vi "Digital_Bridge_3_kart.vi"() -> ()   [LabVIEW 2014]
uses:
  <vilib>/Utility/error.llb/DialogType.ctl
  <vilib>/DAQmx/write.llb/DAQmx Write (Analog 1D Wfm NChan NSamp).vi
  DB_Global_4_kart-Test.vi
  <vilib>/DAQmx/create/channels.llb/DAQmx Create Channel (AO-Voltage-Basic).vi
  <vilib>/DAQmx/configure/timing.llb/DAQmx Timing (Sample Clock).vi
  <vilib>/DAQmx/create/channels.llb/DAQmx Create Channel (AI-Voltage-Basic).vi
  <vilib>/DAQmx/configure/trigger.llb/DAQmx Start Trigger (Digital Edge).vi
  <vilib>/DAQmx/miscellaneous.llb/DAQmx Fill In Error Info.vi
  Sub_VI/show_sensitivity.vi
  First_input_values.vi
  <resource>/objmgr/daqmx.rc
  <vilib>/measure/NI_MABase.lvlib
panel:
  out "input values 2":dbl[](array[numeric])
  out "Y Range KV":dbl
  out "Y Range W":dbl
  out "Y Range 1R":dbl
  out "Y Range 10R":dbl
  out "Y Range AD":dbl
  out "Y 2.input KV":dbl
  out "Y 2.input W":dbl
  out "Y 2.input 1R":dbl
  out "Y 2.input 10R":dbl
  out "Y 2.input AD":dbl
  out "Y 1.input KV":dbl
  out "Y 1.input W":dbl
  out "Y 1.input 1R":dbl
  out "Y 1.input 10R":dbl
  out "Y 1.input AD":dbl
  out "X Range KV":dbl
  out "X Range W":dbl
  out "X Range 1R":dbl
  out "X Range 10R":dbl
  out "X Range AD":dbl
  out "X 2.input KV":dbl
  out "X 2.input W":dbl
  out "X 2.input 1R":dbl
  out "X 2.input 10R":dbl
  out "X 2.input AD":dbl
  out "X 1.input KV":dbl
  out "X 1.input W":dbl
  out "X 1.input 1R":dbl
  out "X 1.input 10R":dbl
  out "X 1.input AD":dbl
  in  "Open all":bool
  in  "Kelvin":bool
  in  "Wagner":bool
  in  "1R":bool
  in  "10R":bool
  in  "AD":bool
  out "count meas":u16
  out "cycle 10r 1r":bool[](array[boolean])
  out "dummy fix default":bool
  out "1 or 10":i32
  in  "read x1 y1":bool
  in  "read x2 y2":bool
  in  "result phase":bool
  in  "read x1 y1 2":bool
  in  "read x2 y2 2":bool
  in  "result phase 2":bool
  in  "read x1 y1 3":bool
  in  "read x2 y2 3":bool
  in  "result phase 3":bool
  in  "read x1 y1 5":bool
  in  "read x2 y2 5":bool
  in  "result phase 5":bool
  in  "result phase 4":bool
  in  "Output Y2":dbl
  in  "Output X2":dbl
  in  "Output Y1":dbl
  in  "Output X1":dbl
  in  "read x2 y2 4":bool
  in  "read x1 y1 4":bool
  in  "Contiune AD":bool
  in  "Contiune Kelvin":bool
  in  "Contiune Wagner":bool
  in  "Contiune 1R":bool
  in  "Contiune 10R":bool
  out "error 2":bool
  out "Outpu Denge Kosulu y1_y2":dbl[][](array[numeric])
  out "Output Denge Kosulu x1_x2":dbl[][](array[numeric])
  out "Output Denge Kosulu x2_y2":dbl[][](array[numeric])
  in  "fix default":bool
  in  "Cluster 2":T1
  in  "Cluster":T2
  out "input values":dbl[](array[numeric])
  out "stop listbox":bool
  out "F Values Array":dbl[][](array[numeric])
  out "extra default values":dbl[][](array[numeric])
  out "control hz array":dbl[][](array[numeric])
  out "Frekanslar":dbl[](array[numeric])
  out "Denge Kosulu y1_y2":dbl[][](array[numeric])
  out "Denge Kosulu x1_x2":dbl[][](array[numeric])
  out "Denge Kosulu x2_y2":dbl[][](array[numeric])
  out "Other Boolean Array":bool[](array[boolean])
  out "Other Array":dbl[](array[numeric])
  out "Kelvin F/P Array":dbl[][](array[numeric])
  out "Wagner F/P Array":dbl[][](array[numeric])
  out "1R F/P Array":dbl[][](array[numeric])
  out "10R F/P Array":dbl[][](array[numeric])
  out "AD F/P Array":dbl[][](array[numeric])
  in  "default input":bool
  out "pass hz":bool
  in  "continue":bool
  out "default values":T3(array[cluster]) {"Kelvin Yk-1" format="%.4p"; "Wagner Yk-1" format="%.4p"; "1R Yk-1" format="%.4p"; "10R Yk-1" format="%.4p"; "Ana Denge Yk-1" format="%.4p"; "Kelvin Yk" format="%.4p"; "Wagner Yk" format="%.4p"; "1R Yk" format="%.4p"; "10R Yk" format="%.4p"; "Ana Denge Yk" format="%.4p"; "Kelvin Xk-1" format="%.4p"; "Wagner Xk-1" format="%.4p"; "1R Xk-1" format="%.4p"; "10R Xk-1" format="%.4p"; "Ana Denge Xk-1" format="%.4p"; "Kelvin Xk" format="%.4p"; "Wagner Xk" format="%.4p"; "1R Xk" format="%.4p"; "10R Xk" format="%.4p"; "Ana Denge Xk" format="%.4p"}
  out "frekans index":dbl
  in  "Direnc 1 [ohm]":dbl=10000.0
  in  "Direnc 2 [ohm]":dbl=1000.0
  in  "error":bool
  out "iterasyon AD":dbl=1.0
  out "first process":bool
  out "reset values":bool
  out "finish":bool
  out "end time":string
  out "start time":string
  out "Iterasyon Successful":dbl
  in  "RESET SENS Y":bool
  in  "RESET SENS X":bool
  in  "RESET SENS Y 5":bool
  in  "RESET SENS X 5":bool
  in  "RESET SENS Y 3":bool
  in  "RESET SENS X 3":bool
  in  "RESET SENS Y 2":bool
  in  "RESET SENS X 2":bool
  in  "RESET SENS Y 4":bool
  in  "RESET SENS X 4":bool
  in  "Activate":bool
  in  "Denge Kolu":u16(ring) items=["Default", "Ana Denge", "Wagner", "10R", "1R"]
  in  "Yedek Kart offset":dbl caption="Offset"
  in  "SWITCH":bool
  in  "Mux2":u16(ring) items=["Wagner", "Ground"]
  in  "Mux1":u16(ring) items=["Open All", "Ana Denge", "10R", "1R"]
  in  "Stop":bool
  in  "GPIB In":refnum<visa-resource-name>="GPIB0::8::INSTR"
  in  "Reference Phase (0.000 degrees)":string
  in  "REFERANS FAZ":bool
  in  "Input Source (0: A)":u16(ring) items=["A", "A-B"]
  in  "INPUT SOURCE":bool
  in  "Sensitivity":u16(ring)=13 items=["2 nV", "5 nV", "10 nV", "20 nV", "50 nV", "100 nV", "200 nV", "500 nV", "1 uV", "2 uV", "5 uV", "10 uV", "20 uV", "50 uV", "100 uV", "200 uV", "500 uV", "1mV", "2 mV", "5 mV", "10 mV", "20 mV", "50 mV", "100 mV", "200 mV", "500 mV", "1 V"]
  in  "SENSITIVITY":bool
  in  "Tab Control":T4(tab)=enum."Wagner"
  in  "Manuel Input":bool
  in  "delay s":u32=2 min=1 max=100
  in  "delay f":u32=2 min=1 max=100
  in  "set":u16=1 min=1 max=100
  in  "BASLAT":bool
  in  "Denge Seçimi":u8=4 min=1 max=5
  in  "Manuel/Otomatik":enum16{"Manuel", "Otomatik"}(ring)=enum."Otomatik"
  out "Hatalar":string[](array[string])
  in  "olcum":u16=1 min=1 max=100
  in  "Frekans Listbox":i32[](listbox)=[12]
  in  "Default Values Listbox":i32[](listbox)=[4]
  in  "Direnc 1 - Direnc 2":u32(ring)=2 items=["1M(Ohm) / 100K(Ohm)", "100K(Ohm) / 10K(Ohm)", "10K(Ohm) / 1K(Ohm)", "1K(Ohm) / 100(Ohm)", "100(Ohm) / 10(Ohm)", "10(Ohm) / 1(Ohm)", "1M(Ohm) / 1M(Ohm)", "100K(Ohm) / 100K(Ohm)", "10K(Ohm) / 10K(Ohm)", "1K(Ohm) / 1K(Ohm)", "100(Ohm) / 100(Ohm)", "10(Ohm) / 10(Ohm)", "1(Ohm) / 1(Ohm)", "1000nF / 100nF (CP)", "100nF / 10nF (CP)", "10nF / 1nF (CP)", "1nF / 100pF (CP)", "100pF / 10pF (CP)", "10pF / 1pF (CP)", "1000nF / 1000nF (CP)", "100nF / 100nF (CP)", "10nF / 10nF (CP)", "1nF / 1nF (CP)", "100pF / 100pF (CP)", "10pF / 10pF (CP)", "1pF / 1pF (CP)"]
  in  "Multicolumn Listbox":i32(listbox)
  in  "Cp - 10R":u16(ring) items=["1nF", "10nF", "100nF", "1uF", "10uF"]
  in  "Cp - 1R":u16(ring) items=["1nF", "10nF", "100nF", "1uF", "10uF"]
  in  "value 10R":u16
  in  "value 1R":u16
  in  "Sheet name":string="10k1k"
  in  "Manuel Setup":bool
  in  "interrupt":bool=TRUE
  in  "START X":bool
  in  "START Y":bool
  out "AD X(k-1)":dbl=0.01
  out "AD Xk":dbl
  out "AD Yk":dbl
  out "AD Y(k-1)":dbl=0.01
  in  "AD X_1":dbl=3e-06
  in  "AD X_2":dbl=4e-07
  in  "AD Y_1":dbl=3e-06
  in  "AD Y_2":dbl=4e-07
  out "İterasyon X":dbl
  out "İterasyon Y":dbl
  in  "X":bool
  in  "X1":bool
  in  "RANGE KONTROL X":bool
  in  "IF ELSE X":bool
  in  "KONTROL Y":bool
  out "result output x [AD]":dbl
  out "output 2 x [ana denge]":dbl
  out "output 1 x [ana denge]":dbl
  out "input 1 x [ana denge]":dbl format="%.4p"
  out "input 2 x [ana denge]":dbl format="%.4p"
  in  "Y1":bool
  in  "Y":bool
  in  "IF ELSE Y":bool
  in  "RANGE KONTROL Y":bool
  in  "KONTROL X":bool
  out "result output y [AD]":dbl
  out "input 1 y [ana denge]":dbl format="%.4p"
  out "input 2 y [ana denge]":dbl format="%.4p"
  out "output 1 y [ana denge]":dbl
  out "output 2 y [ana denge]":dbl
  in  "PASS ANA D":bool
  out "Boolean":bool
  in  "Ana denge Switch":bool
  in  "Start AD Y":bool
  in  "Start AD X":bool
  in  "auto phase AD":bool
  in  "Reserve AD":u16(ring) items=["Max", "Manuel", "Min"]
  in  "Optimum Range 1":bool
  in  "START X 2":bool
  in  "START Y 2":bool
  out "İterasyon Y 2":dbl
  out "İterasyon X 2":dbl
  out "10R Y(k-1)":dbl=3.0
  out "10R Yk":dbl
  out "10R X(k-1)":dbl=3.0
  out "10R Xk":dbl
  in  "10R  Y_1":dbl=4e-05
  in  "10R X_1":dbl=4e-05
  in  "10R Y_2":dbl=2e-05
  in  "10R X_2":dbl=2e-05
  in  "X 2":bool
  in  "X1 2":bool
  in  "RANGE KONTROL X 2":bool
  in  "IF ELSE X 2":bool
  in  "KONTROL Y 2":bool
  out "result output x [10R]":dbl
  out "output 2 x [10R]":dbl
  out "output 1 x [10R]":dbl
  out "input 1 x [10R]":dbl format="%.4p"
  out "input 2 x [10R]":dbl format="%.4p"
  in  "Y 2":bool
  in  "Y1 2":bool
  in  "IF ELSE Y 2":bool
  in  "RANGE KONTROL Y 2":bool
  in  "KONTROL X 2":bool
  out "result output y [10R]":dbl
  out "input 1 y [10R]":dbl format="%.4p"
  out "input 2 y [10R]":dbl format="%.4p"
  out "output 1 y [10R]":dbl
  out "output 2 y [10R]":dbl
  in  "PASS 10R":bool
  in  "10R switch":bool
  in  "Start 10R Y":bool
  in  "Start 10R X":bool
  out "Boolean 2":bool
  in  "auto phase 10R":bool
  in  "Reserve 10R":u16(ring) items=["Max", "Manuel", "Min"]
  in  "Optimum Range 2":bool
  in  "START X 3":bool
  in  "START Y 3":bool
  out "İterasyon Y 3":dbl
  out "İterasyon X 3":dbl
  out "1R Y(k-1)":dbl=2.0
  out "1R Yk":dbl
  out "1R X(k-1)":dbl=2.0
  out "1R Xk":dbl
  in  "1R Y_1":dbl=4e-05
  in  "1R X_1":dbl=4e-05
  in  "1R Y_2":dbl=2e-05
  in  "1R X_2":dbl=2e-05
  in  "X 3":bool
  in  "X1 3":bool
  in  "RANGE KONTROL X 3":bool
  in  "IF ELSE X 3":bool
  in  "KONTROL Y 3":bool
  out "result output x [1R]":dbl
  out "output 2 x [1R]":dbl
  out "output 1 x [1R]":dbl
  out "input 1 x [1R]":dbl format="%.4p"
  out "input 2 x [1R]":dbl format="%.4p"
  in  "Y 3":bool
  in  "Y1 3":bool
  in  "IF ELSE Y 3":bool
  in  "RANGE KONTROL Y 3":bool
  in  "KONTROL X 3":bool
  out "result output y [1R]":dbl
  out "input 1 y [1R]":dbl format="%.4p"
  out "input 2 y [1R]":dbl format="%.4p"
  out "output 1 y [1R]":dbl
  out "output 2 y [1R]":dbl
  in  "PASS 1R":bool
  in  "1R switch":bool
  in  "Start 1R Y":bool
  in  "Start 1R X":bool
  out "Boolean 3":bool
  in  "auto phase 1R":bool
  in  "Reserve 1R":u16(ring) items=["Max", "Manuel", "Min"]
  in  "Optimum Range 3":bool
  in  "START X 4":bool
  in  "START Y 4":bool
  out "İterasyon Y 4":dbl
  out "İterasyon X 4":dbl
  out "Wagner Y(k-1)":dbl=0.1
  out "Wagner Yk":dbl
  out "Wagner  X(k-1)":dbl=0.1
  out "Wagner Xk":dbl
  in  "Wagner Y_1":dbl=5e-05
  in  "Wagner X_1":dbl=5e-05
  in  "Wagner Y_2":dbl=2e-05
  in  "Wagner X_2":dbl=2e-05
  out "result output x [Wagner]":dbl
  out "output 2 x [wagner]":dbl
  out "output 1 x [wagner]":dbl
  in  "X 4":bool
  in  "X1 4":bool
  out "input 1 x [wagner]":dbl format="%.4p"
  out "input 2 x [wagner]":dbl format="%.4p"
  in  "RANGE KONTROL X 4":bool
  in  "IF ELSE X 4":bool
  in  "KONTROL Y 4":bool
  in  "PASS WAGNER":bool
  out "result output y [Wagner]":dbl
  out "input 1 y [wagner]":dbl format="%.4p"
  out "input 2 y [wagner]":dbl format="%.4p"
  out "output 1 y [wagner]":dbl
  out "output 2 y [wagner]":dbl
  in  "IF ELSE Y 4":bool
  in  "RANGE KONTROL Y 4":bool
  in  "Y 4":bool
  in  "Y1 4":bool
  in  "KONTROL X 4":bool
  in  "wagner switch":bool
  in  "Start Wagner Y":bool
  in  "Start Wagner X":bool
  out "Boolean 4":bool
  in  "auto phase wagner":bool
  in  "Reserve Wagner":u16(ring) items=["Max", "Manuel", "Min"]
  in  "Optimum Range 4":bool
  in  "START X 5":bool
  in  "START Y 5":bool
  out "İterasyon Y 5":dbl
  out "İterasyon X 5":dbl
  out "Kelvin Y(k-1)":dbl=0.01
  out "Kelvin Yk":dbl
  out "Kelvin X(k-1)":dbl=0.01
  out "Kelvin Xk":dbl
  in  "Kelvin Y_1":dbl=3e-06
  in  "Kelvin X_1":dbl=3e-06
  in  "Kelvin Y_2":dbl=2e-07
  in  "Kelvin X_2":dbl=2e-07
  in  "X 5":bool
  in  "X1 5":bool
  in  "RANGE KONTROL X 5":bool
  in  "IF ELSE X 5":bool
  in  "KONTROL Y 5":bool
  out "result output x [Kelvin]":dbl
  out "output 2 x [kelvin]":dbl
  out "output 1 x [kelvin]":dbl
  out "input 1 x [kelvin]":dbl format="%.4p"
  out "input 2 x [kelvin]":dbl format="%.4p"
  in  "Y 5":bool
  in  "Y1 5":bool
  in  "IF ELSE Y 5":bool
  in  "RANGE KONTROL Y 5":bool
  in  "KONTROL X 5":bool
  out "result output y [Kelvin]":dbl
  out "input 1 y [kelvin]":dbl format="%.4p"
  out "input 2 y [kelvin]":dbl format="%.4p"
  out "output 1 y [kelvin]":dbl
  out "output 2 y [kelvin]":dbl
  in  "PASS KELVIN":bool
  in  "kelvin switch":bool
  in  "Start Kelvin Y":bool
  in  "Start Kelvin X":bool
  out "Boolean 5":bool
  in  "auto phase kelvin":bool
  in  "Reserve Kelvin":u16(ring) items=["Max", "Manuel", "Min"]
  in  "Optimum Range 5":bool
  out "iterasyon KELVIN":dbl=1.0
  out "iterasyon WAGNER":dbl
  out "iterasyon 1R":dbl=1.0
  out "iterasyon 10R":dbl=1.0
  # "Eski Sistem"
  # "Ölçeceğiniz dirençlerin değerlerini seçiniz\nCp değerlerini seçmeyi ve uygulamayı unutmayınız"
  # "Tüm dengeleri dengelesin istiyorsanız otomatik,\nistediğiniz dengeyi dengelemek istiyorsanız manuel seçiniz"
  # "Hatalar"
  # "1. Ana denge \\ 2. 10R \\ 3. 1R \\ 4. Wagner \\ 5. Kelvin"
  # "Excel'den hazır olarak \nalabileceğiniz değerler var ise seçiniz"
  # "Frekans'a göre denge koşulu değiştirmek için ilgili yeri doldurunuz\nNot: AD -> Ana denge | W -> Wagner | K -> Kelvin"
  # "Frekans seçimi"
  # "Shift + yön tuşları ile hücreleri gezebilirsiniz"
  # "Excelden aldığınız frekans verisinin denge koşulunu değiştirmek istemiyorsanız\n\"Interrupt\" butonu pasif hale getiriniz"
  # "X ve Y iterasyon değerleri"
  # "X ve Y koşul değerleri"
  # "Başlatma butonları"
  # "Ön kontrol merkezi"
  # "X ve Y denge değerleri"
  # "X kontrol merkezi"
  # "Y kontrol merkezi"
  # "X ve Y iterasyon değerleri"
  # "X ve Y koşul değerleri"
  # "Başlatma butonları"
  # "Ön kontrol merkezi"
  # "X ve Y denge değerleri"
  # "X kontrol merkezi"
  # "Y kontrol merkezi"
  # "X ve Y koşul değerleri"
  # "X ve Y iterasyon değerleri"
  # "Başlatma butonları"
  # "Ön kontrol merkezi"
  # "X ve Y denge değerleri"
  # "X kontrol merkezi"
  # "Y kontrol merkezi"
  # "X ve Y iterasyon değerleri"
  # "X ve Y koşul değerleri"
  # "Başlatma butonları"
  # "Ön kontrol merkezi"
  # "X ve Y denge değerleri"
  # "X kontrol merkezi"
  # "Y kontrol merkezi"
  # "X ve Y koşul değerleri"
  # "X ve Y iterasyon değerleri"
  # "Başlatma butonları"
  # "Ön kontrol merkezi"
  # "X ve Y denge değerleri"
  # "X kontrol merkezi"
  # "Y kontrol merkezi"
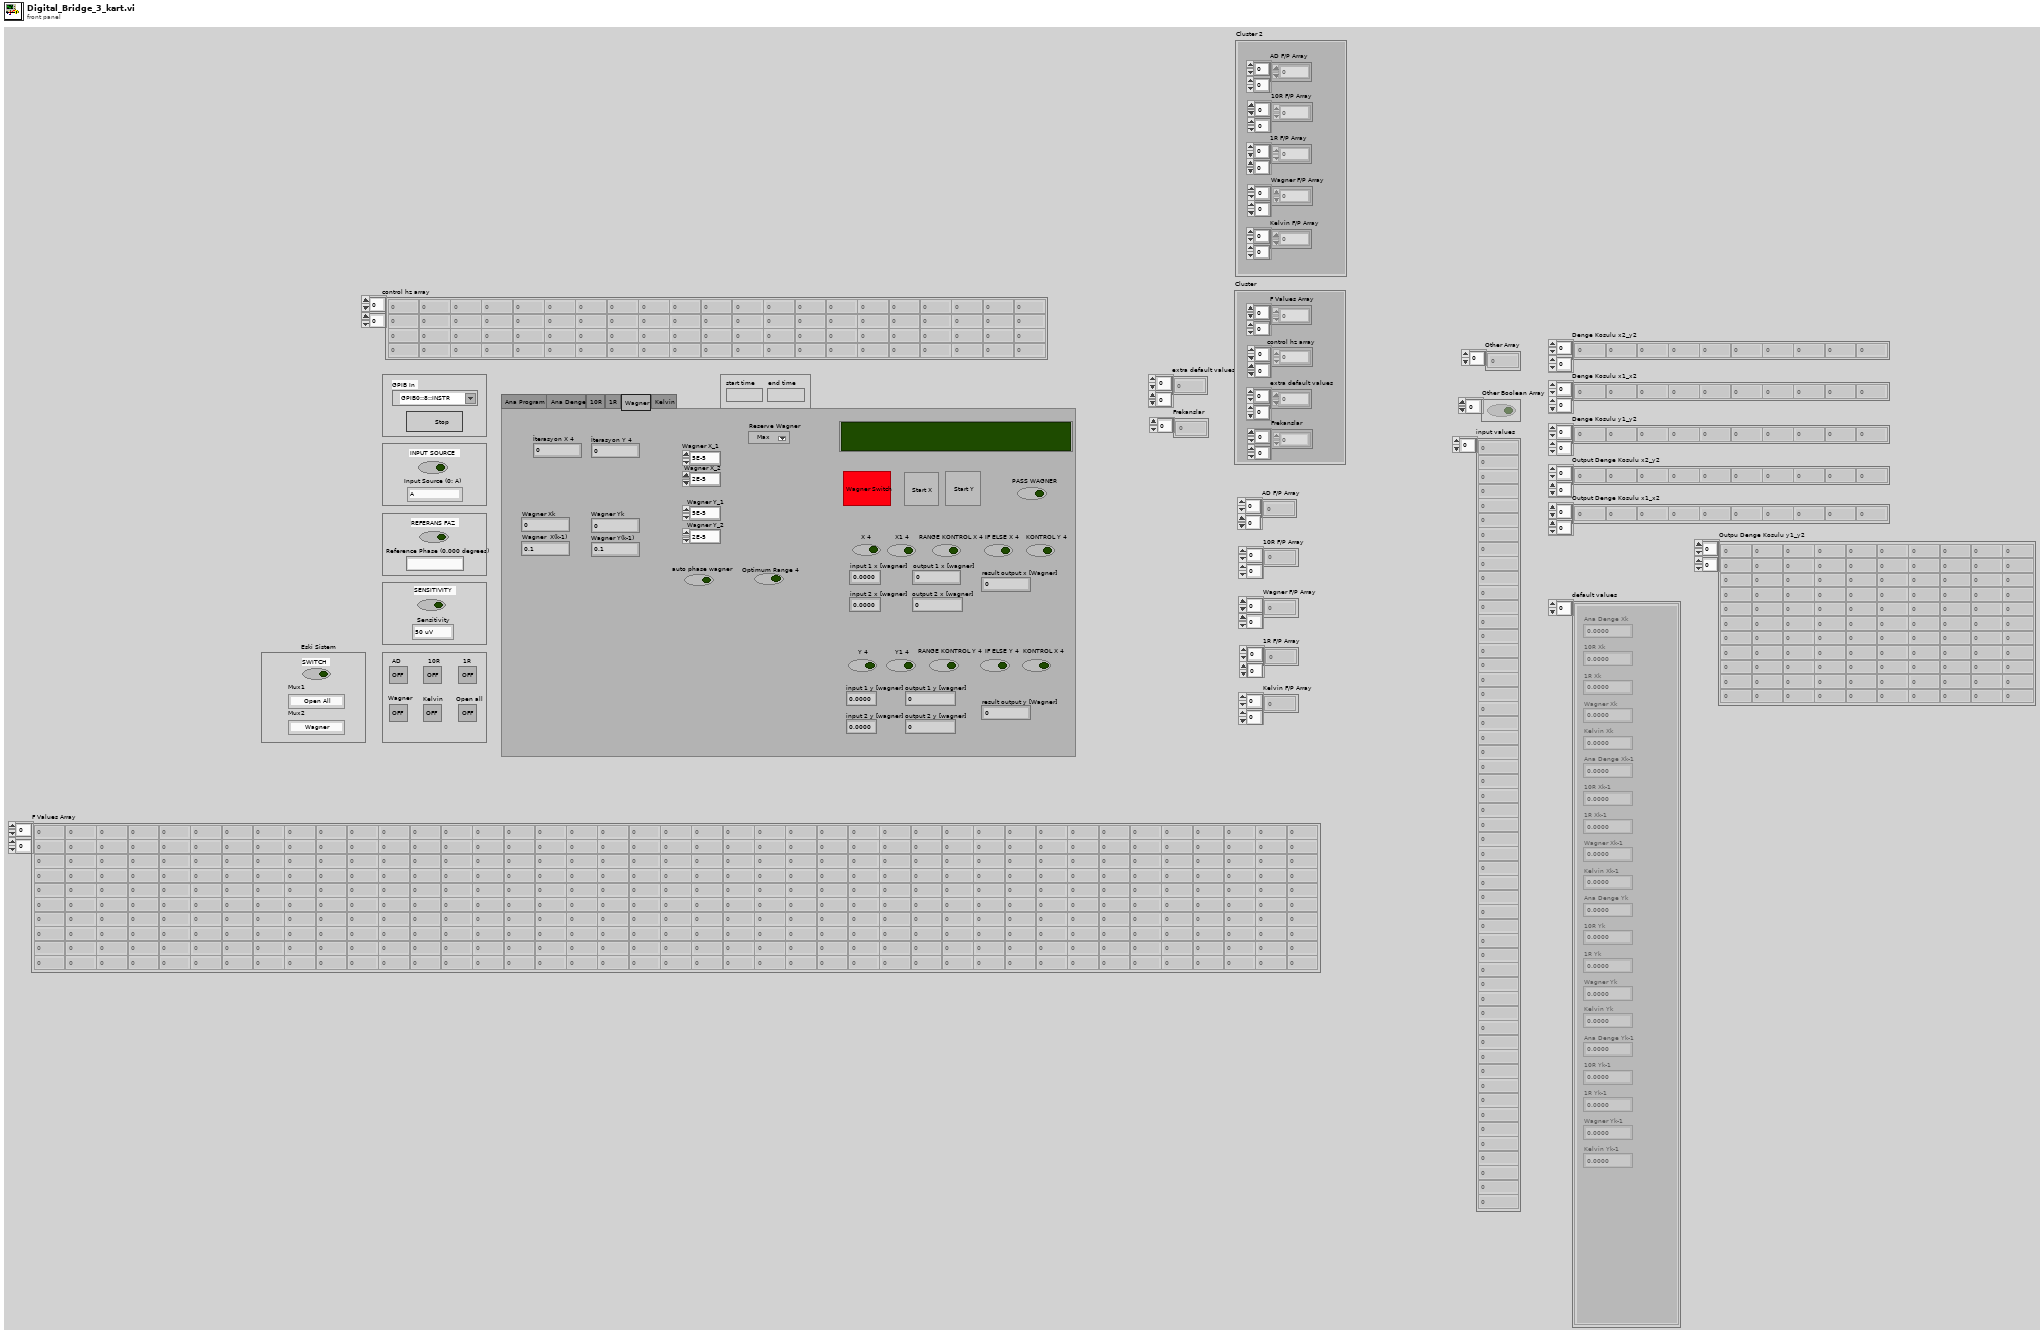
[diagram p1: front panel]
types:
  T1 = cluster{"AD F/P Array":dbl[][], "10R F/P Array":dbl[][], "1R F/P Array":dbl[][], "Wagner F/P Array":dbl[][], "Kelvin F/P Array":dbl[][]}
  T2 = cluster{"F Values Array":dbl[][], "control hz array":dbl[][], "extra default values":dbl[][], "Frekanslar":dbl[][]}
  T3 = cluster{"Ana Denge Xk":dbl, "10R Xk ":dbl, "1R Xk ":dbl, "Wagner Xk":dbl, "Kelvin Xk ":dbl, "Ana Denge Xk-1":dbl, "10R Xk-1":dbl, "1R Xk-1":dbl, "Wagner Xk-1":dbl, "Kelvin Xk-1":dbl, "Ana Denge Yk":dbl, "10R Yk ":dbl, "1R Yk ":dbl, "Wagner Yk ":dbl, "Kelvin Yk  ":dbl, "Ana Denge Yk-1":dbl, "10R Yk-1":dbl, "1R Yk-1":dbl, "Wagner Yk-1":dbl, "Kelvin Yk-1":dbl}[]
  T4 = enum32{"Ana Program", "Ana Denge", "10R", "1R", "Wagner", "Kelvin"}
  T5 = enum8{"Enabled", "Disabled", "Disabled and Grayed Out"}
  T6 = typedef "DialogType.ctl" = u16
  T7 = enum16{"Sine Wave", "Triangle Wave", "Square Wave", "Sawtooth Wave"}
  T8 = typedef "LVPoint32TypeDef.ctl" = cluster{"Horizontal":i32, "Vertical":i32}
  T9 = typedef "LVRowAndColumnTypeDef.ctl" = cluster{"Row":i32, "Column":i32}
  T10 = cluster{"Ana Denge Xk":dbl, "Wagner Xk":dbl, "10R Xk":dbl, "1R Xk":dbl, "Kelvin Xk":dbl, "Ana Denge Xk-1":dbl, "Wagner Xk-1":dbl, "10R Xk-1":dbl, "1R Xk-1":dbl, "Kelvin Xk-1":dbl, "Ana Denge Yk":dbl, "Wagner Yk":dbl, "10R Yk":dbl, "1R Yk":dbl, "Kelvin Yk":dbl, "Ana Denge Yk-1":dbl, "Wagner Yk-1":dbl, "10R Yk-1":dbl, "1R Yk-1":dbl, "Kelvin Yk-1":dbl}[]
  T11 = cluster{"Ana Denge Xk":dbl, "10R Xk":dbl, "1R Xk":dbl, "Wagner Xk":dbl, "Kelvin Xk":dbl, "Ana Denge Xk-1":dbl, "10R Xk-1":dbl, "1R Xk-1":dbl, "Wagner Xk-1":dbl, "Kelvin Xk-1":dbl, "Ana Denge Yk":dbl, "10R Yk":dbl, "1R Yk":dbl, "Wagner Yk":dbl, "Kelvin Yk":dbl, "Ana Denge Yk-1":dbl, "10R Yk-1":dbl, "1R Yk-1":dbl, "Wagner Yk-1":dbl, "Kelvin Yk-1":dbl}[]
  T12 = cluster{"Ana Denge Xk":dbl, "10R Xk ":dbl, "1R Xk ":dbl, "Wagner Xk":dbl, "Kelvin Xk ":dbl, "Ana Denge Xk-1":dbl, "10R Xk-1":dbl, "1R Xk-1":dbl, "Wagner Xk-1":dbl, "Kelvin Xk-1":dbl, "Ana Denge Yk":dbl, "10R Yk ":dbl, "1R Yk ":dbl, "Wagner Yk ":dbl, "Kelvin Yk  ":dbl, "Ana Denge Yk-1":dbl, "10R Yk-1":dbl, "1R Yk-1":dbl, "Wagner Yk-1":dbl, "Kelvin Yk-1":dbl}
diagram:
  n1 = flat-sequence {
    frame #0 {
      n2 = flat-sequence {
        frame #0 {
          w20 = FALSE ("Boolean 5")
          w21 = FALSE
          w23 = FALSE
          w24 = FALSE ("Boolean 5")
          w22 = FALSE ("Boolean 5")
          w25 = 0.0 ("amplitude 2/0")
          w26 = FALSE
          w27 = FALSE
          n3 = local write "PASS 10R"(w27) -> ()
          n4 = local write "PASS 1R"(w27) -> ()
          n5 = local write "PASS ANA D"(w27) -> ()
          n6 = local write "PASS KELVIN"(w27) -> ()
          n7 = local write "PASS WAGNER"(w27) -> ()
          n8 = local write "Ana denge Switch"(w23) -> ()
          n9 = local write "Start AD X"(w23) -> ()
          n10 = local write "Start AD Y"(w23) -> ()
          n11 = local write "10R switch"(w23) -> ()
          n12 = local write "Start 10R X"(w23) -> ()
          n13 = local write "Start 10R Y"(w23) -> ()
          n14 = local write "1R switch"(w23) -> ()
          n15 = local write "Start 1R X"(w23) -> ()
          n16 = local write "Start 1R Y"(w23) -> ()
          n17 = local write "wagner switch"(w23) -> ()
          n18 = local write "Start Wagner X"(w23) -> ()
          n19 = local write "Start Wagner Y"(w23) -> ()
          n20 = local write "kelvin switch"(w23) -> ()
          n21 = local write "Start Kelvin X"(w23) -> ()
          n22 = local write "Start Kelvin Y"(w23) -> ()
          n23 = global write "DB_Global_4_kart-Test.vi" "amplitude 2/0"(w25) -> ()
          n24 = global write "DB_Global_4_kart-Test.vi" "phase 2/ 0"(w25) -> ()
          n25 = global write "DB_Global_4_kart-Test.vi" "amplitude 3/0"(w25) -> ()
          n26 = global write "DB_Global_4_kart-Test.vi" "phase 3/0"(w25) -> ()
          n27 = global write "DB_Global_4_kart-Test.vi" "amplitude 1/1"(w25) -> ()
          n28 = global write "DB_Global_4_kart-Test.vi" "phase 1/1"(w25) -> ()
          n29 = global write "DB_Global_4_kart-Test.vi" "amplitude 2/1"(w25) -> ()
          n30 = global write "DB_Global_4_kart-Test.vi" "phase 2/1"(w25) -> ()
          n31 = global write "DB_Global_4_kart-Test.vi" "amplitude 3/1"(w25) -> ()
          n32 = global write "DB_Global_4_kart-Test.vi" "phase 3/1"(w25) -> ()
          n33 = local write "Boolean"(w22) -> ()
          n34 = local write "Boolean 2"(w22) -> ()
          n35 = local write "Boolean 3"(w22) -> ()
          n36 = local write "Boolean 4"(w22) -> ()
          n37 = local write "Boolean 5"(w22) -> ()
          n38 = local write "KONTROL Y"(w26) -> ()
          n39 = local write "KONTROL X"(w26) -> ()
          n40 = local write "KONTROL Y 5"(w26) -> ()
          n41 = local write "KONTROL X 5"(w26) -> ()
          n42 = local write "KONTROL Y 3"(w26) -> ()
          n43 = local write "KONTROL X 2"(w26) -> ()
          n44 = local write "KONTROL Y 2"(w26) -> ()
          n45 = local write "KONTROL X 3"(w26) -> ()
          n46 = local write "KONTROL Y 4"(w26) -> ()
          n47 = local write "KONTROL X 4"(w26) -> ()
          n48 = local write "X"(w26) -> ()
          n49 = local write "RANGE KONTROL X 5"(w26) -> ()
          n50 = local write "Y"(w26) -> ()
          n51 = local write "RANGE KONTROL X 2"(w26) -> ()
          n52 = local write "X 2"(w26) -> ()
          n53 = local write "RANGE KONTROL X 3"(w26) -> ()
          n54 = local write "Y 2"(w26) -> ()
          n55 = local write "RANGE KONTROL Y 5"(w26) -> ()
          n56 = local write "X 3"(w26) -> ()
          n57 = local write "RANGE KONTROL Y"(w26) -> ()
          n58 = local write "Y 3"(w26) -> ()
          n59 = local write "read x1 y1"(w21) -> ()
          n60 = local write "read x2 y2"(w21) -> ()
          n61 = local write "result phase"(w21) -> ()
          n62 = local write "read x1 y1 2"(w21) -> ()
          n63 = local write "read x2 y2 2"(w21) -> ()
          n64 = local write "result phase 2"(w21) -> ()
          n65 = local write "read x1 y1 3"(w21) -> ()
          n66 = local write "read x2 y2 3"(w21) -> ()
          n67 = local write "result phase 3"(w21) -> ()
          n68 = local write "read x1 y1 4"(w21) -> ()
          n69 = local write "read x2 y2 4"(w21) -> ()
          n70 = local write "result phase 4"(w21) -> ()
          n71 = local write "read x1 y1 5"(w21) -> ()
          n72 = local write "read x2 y2 5"(w21) -> ()
          n73 = local write "result phase 5"(w21) -> ()
          n74 = local write "X1"(w26) -> ()
          n75 = local write "IF ELSE X 5"(w26) -> ()
          n76 = local write "Y1"(w26) -> ()
          n77 = local write "IF ELSE Y 4"(w26) -> ()
          n78 = local write "X1 2"(w26) -> ()
          n79 = local write "IF ELSE Y 5"(w26) -> ()
          n80 = local write "Y1 2"(w26) -> ()
          n81 = local write "IF ELSE Y"(w26) -> ()
          n82 = local write "X1 3"(w26) -> ()
          n83 = local write "IF ELSE X"(w26) -> ()
          n84 = local write "Y1 3"(w26) -> ()
          n85 = local write "RANGE KONTROL X"(w26) -> ()
          n86 = local write "X 4"(w26) -> ()
          n87 = local write "RANGE KONTROL Y 2"(w26) -> ()
          n88 = local write "RANGE KONTROL Y 3"(w26) -> ()
          n89 = local write "X 5"(w26) -> ()
          n90 = local write "RANGE KONTROL X 4"(w26) -> ()
          n91 = local write "Y 5"(w26) -> ()
          n92 = local write "RANGE KONTROL Y 4"(w26) -> ()
          n93 = local write "Y 4"(w26) -> ()
          n94 = local write "auto phase AD"(w24) -> ()
          n95 = local write "auto phase 10R"(w24) -> ()
          n96 = local write "auto phase 1R"(w24) -> ()
          n97 = local write "auto phase wagner"(w24) -> ()
          n98 = local write "auto phase kelvin"(w24) -> ()
          n99 = local write "Optimum Range 1"(w20) -> ()
          n100 = local write "Optimum Range 2"(w20) -> ()
          n101 = local write "Optimum Range 3"(w20) -> ()
          n102 = local write "Optimum Range 4"(w20) -> ()
          n103 = local write "Optimum Range 5"(w20) -> ()
          n104 = local write "fix default"(FALSE ("Optimum Range 5")) -> ()
          n105 = local write "IF ELSE Y 2"(w26) -> ()
          n106 = local write "X1 4"(w26) -> ()
          n107 = local write "IF ELSE X 2"(w26) -> ()
          n108 = local write "Y1 4"(w26) -> ()
          n109 = local write "IF ELSE Y 3"(w26) -> ()
          n110 = local write "X1 5"(w26) -> ()
          n111 = local write "IF ELSE X 3"(w26) -> ()
          n112 = local write "Y1 5"(w26) -> ()
          n113 = local write "IF ELSE X 4"(w26) -> ()
        }
      }
      n114 = local write "BASLAT"(FALSE ("BASLAT")) -> ()
      n115 = local write "Stop"(FALSE ("Stop")) -> ()
      n116 = property on="Multicolumn Listbox" class="MCListbox (strict)"("Allow Editing Cells"=TRUE) -> ()  [unwired: 2 in, 2 out]
      n117 = property on="Frekans Listbox" class="LstBox (strict)"("DisabledEnum"=T5."Enabled" ("Disabled")) -> ()  [unwired: 2 in, 2 out]
      n118 = property on="Default Values Listbox" class="LstBox (strict)"("DisabledEnum"=T5."Enabled" ("Disabled")) -> ()  [unwired: 2 in, 2 out]
      n119 = Initialize Array(FALSE, 1 ("dimension size")) -> (→"cycle 10r 1r":bool[])
      "finish" <- FALSE ("finish")
      "reset values" <- FALSE ("reset values")
      "first process" <- TRUE ("first process")
      "pass hz" <- FALSE ("pass hz")
      "stop listbox" <- FALSE ("pass hz 2")
      "error 2" <- FALSE ("error 2")
      "dummy fix default" <- TRUE ("dummy fix default")
      "end time" <- "" ("end time")
      "start time" <- "" ("start time")
      "count meas" <- u16 0 ("count meas")
    }
    frame #1 {
      n120 = Wait (ms)(milliseconds to wait=u32 1000) -> ()  [unwired: 1 out]
    }
    frame #2 {
      w29 = T6 3 items=["no dialog", "OK message", "continue or stop message", "OK message + warnings", "continue/stop + warnings"] ("type of dialog (OK msg:1)")
      w58 = tag "PXI_Clk10" ("RefClk.Src")
      w138 = 10.0  # timeout (s)
      w139 = FALSE  # auto start
      w145 = 10.0  # timeout (s)
      w144 = FALSE  # auto start
      w150 = 10097 items=["Allow Regeneration"=10097, "Do Not Allow Regeneration"=10158]  # regeneration mode
      w152 = 10123 items=["Finite Samples"=10178, "Continuous Samples"=10123, "Hardware Timed Single Point"=12522]  # sample mode
      w153 = 2000  # number of samples
      w154 = 204800.0  # rate
      w157 = 10106 items=["Default"=-1, "RSE"=10083, "Differential"=10106, "Pseudodifferential"=12529]  # output terminal configuration
      w158 = 10348 items=["Volts"=10348, "From Custom Scale"=10065]  # units
      w159 = "VoltageOut_1"  # channel name
      w161 = ""  # custom scale name
      w162 = -10.0  # minimum value
      w163 = 10.0  # maximum value
      (unwired) "Dev1/ao1"  # physical channel
      w165 = 10106 items=["Default"=-1, "RSE"=10083, "Differential"=10106, "Pseudodifferential"=12529]  # output terminal configuration
      w166 = 10348 items=["Volts"=10348, "From Custom Scale"=10065]  # units
      w167 = "VoltageOut_0"  # channel name
      w169 = ""  # custom scale name
      w170 = -10.0  # minimum value
      w171 = 10.0  # maximum value
      (unwired) "Dev1/ao0"  # physical channel
      w173 = TRUE  # auto cleanup
      w199 = 10097 items=["Allow Regeneration"=10097, "Do Not Allow Regeneration"=10158]  # regeneration mode
      w197 = 10123 items=["Finite Samples"=10178, "Continuous Samples"=10123, "Hardware Timed Single Point"=12522]  # sample mode
      w196 = 2000  # number of samples
      w195 = 204800.0  # rate
      w192 = 10106 items=["Default"=-1, "RSE"=10083, "Differential"=10106, "Pseudodifferential"=12529]  # output terminal configuration
      w191 = 10348 items=["Volts"=10348, "From Custom Scale"=10065]  # units
      w190 = "VoltageOut_1"  # channel name
      w188 = ""  # custom scale name
      w187 = -10.0  # minimum value
      w186 = 10.0  # maximum value
      (unwired) "Dev1/ao1"  # physical channel
      w184 = 10106 items=["Default"=-1, "RSE"=10083, "Differential"=10106, "Pseudodifferential"=12529]  # output terminal configuration
      w183 = 10348 items=["Volts"=10348, "From Custom Scale"=10065]  # units
      w182 = "VoltageOut_0"  # channel name
      w180 = ""  # custom scale name
      w179 = -10.0  # minimum value
      w178 = 10.0  # maximum value
      (unwired) "Dev1/ao0"  # physical channel
      w176 = TRUE  # auto cleanup
      w122 = cluster{"Fs":dbl, "#s":dbl} {"Fs"=204800.0, "#s"=20480.0} ("sampling info")
      w123 = T7."Sine Wave" ("signal type")
      w59 = 10000000.0 ("RefClk.Rate")
      w210 = 10.0  # timeout (s)
      w211 = FALSE  # auto start
      w216 = 10097 items=["Allow Regeneration"=10097, "Do Not Allow Regeneration"=10158]  # regeneration mode
      w218 = 10123 items=["Finite Samples"=10178, "Continuous Samples"=10123, "Hardware Timed Single Point"=12522]  # sample mode
      w219 = 2000  # number of samples
      w220 = 204800.0  # rate
      w223 = 10106 items=["Default"=-1, "RSE"=10083, "Differential"=10106, "Pseudodifferential"=12529]  # output terminal configuration
      w224 = 10348 items=["Volts"=10348, "From Custom Scale"=10065]  # units
      w225 = "VoltageOut_1"  # channel name
      w227 = ""  # custom scale name
      w228 = -10.0  # minimum value
      w229 = 10.0  # maximum value
      (unwired) "Dev2/ao1"  # physical channel
      w231 = 10106 items=["Default"=-1, "RSE"=10083, "Differential"=10106, "Pseudodifferential"=12529]  # output terminal configuration
      w232 = 10348 items=["Volts"=10348, "From Custom Scale"=10065]  # units
      w233 = "VoltageOut_0"  # channel name
      w235 = ""  # custom scale name
      w236 = -10.0  # minimum value
      w237 = 10.0  # maximum value
      (unwired) "Dev2/ao0"  # physical channel
      w239 = TRUE  # auto cleanup
      w245 = 10123 items=["Finite Samples"=10178, "Continuous Samples"=10123, "Hardware Timed Single Point"=12522]  # sample mode
      w246 = 2000  # number of samples
      w247 = 204800.0  # rate
      w251 = 10045 items=["AC"=10045, "DC"=10050, "GND"=10066]  # Coupling
      w252 = "Voltage_1"  # ActiveChan
      w255 = 10045 items=["AC"=10045, "DC"=10050, "GND"=10066]  # Coupling
      w256 = "Voltage_0"  # ActiveChan
      w257 = 10106 items=["default"=-1, "RSE"=10083, "NRSE"=10078, "Differential"=10106, "Pseudodifferential"=12529]  # input terminal configuration
      w258 = 10348 items=["Volts"=10348, "From Custom Scale"=10065]  # units
      w259 = "Voltage_1"  # channel name
      w241 = ""  # custom scale name
      w261 = -10.0  # minimum value
      w262 = 10.0  # maximum value
      (unwired) "Dev3/ai1"  # physical channel
      w264 = 10106 items=["default"=-1, "RSE"=10083, "NRSE"=10078, "Differential"=10106, "Pseudodifferential"=12529]  # input terminal configuration
      w265 = 10348 items=["Volts"=10348, "From Custom Scale"=10065]  # units
      w266 = "Voltage_0"  # channel name
      w243 = ""  # custom scale name
      w268 = -10.0  # minimum value
      w269 = 10.0  # maximum value
      (unwired) "Dev3/ai0"  # physical channel
      w271 = TRUE  # auto cleanup
      w300 = 10123 items=["Finite Samples"=10178, "Continuous Samples"=10123, "Hardware Timed Single Point"=12522]  # sample mode
      w299 = 2000  # number of samples
      w298 = 204800.0  # rate
      w294 = 10045 items=["AC"=10045, "DC"=10050, "GND"=10066]  # Coupling
      w293 = "Voltage_1"  # ActiveChan
      w290 = 10045 items=["AC"=10045, "DC"=10050, "GND"=10066]  # Coupling
      w289 = "Voltage_0"  # ActiveChan
      w288 = 10106 items=["default"=-1, "RSE"=10083, "NRSE"=10078, "Differential"=10106, "Pseudodifferential"=12529]  # input terminal configuration
      w287 = 10348 items=["Volts"=10348, "From Custom Scale"=10065]  # units
      w286 = "Voltage_1"  # channel name
      w242 = ""  # custom scale name
      w284 = -10.0  # minimum value
      w283 = 10.0  # maximum value
      (unwired) "Dev2/ai1"  # physical channel
      w281 = 10106 items=["default"=-1, "RSE"=10083, "NRSE"=10078, "Differential"=10106, "Pseudodifferential"=12529]  # input terminal configuration
      w280 = 10348 items=["Volts"=10348, "From Custom Scale"=10065]  # units
      w279 = "Voltage_0"  # channel name
      w244 = ""  # custom scale name
      w277 = -10.0  # minimum value
      w276 = 10.0  # maximum value
      (unwired) "Dev2/ai0"  # physical channel
      w274 = TRUE  # auto cleanup
      w301 = 10123 items=["Finite Samples"=10178, "Continuous Samples"=10123, "Hardware Timed Single Point"=12522]  # sample mode
      w302 = 2000  # number of samples
      w303 = 204800.0  # rate
      w307 = 10045 items=["AC"=10045, "DC"=10050, "GND"=10066]  # Coupling
      w308 = "Voltage_1"  # ActiveChan
      w311 = 10045 items=["AC"=10045, "DC"=10050, "GND"=10066]  # Coupling
      w312 = "Voltage_0"  # ActiveChan
      w313 = 10106 items=["default"=-1, "RSE"=10083, "NRSE"=10078, "Differential"=10106, "Pseudodifferential"=12529]  # input terminal configuration
      w314 = 10348 items=["Volts"=10348, "From Custom Scale"=10065]  # units
      w315 = "Voltage_1"  # channel name
      w317 = ""  # custom scale name
      w318 = -10.0  # minimum value
      w319 = 10.0  # maximum value
      (unwired) "Dev1/ai1"  # physical channel
      w321 = 10106 items=["default"=-1, "RSE"=10083, "NRSE"=10078, "Differential"=10106, "Pseudodifferential"=12529]  # input terminal configuration
      w322 = 10348 items=["Volts"=10348, "From Custom Scale"=10065]  # units
      w323 = "Voltage_0"  # channel name
      w325 = ""  # custom scale name
      w326 = -10.0  # minimum value
      w327 = 10.0  # maximum value
      (unwired) "Dev1/ai0"  # physical channel
      w329 = TRUE  # auto cleanup
      # "excel den alırken direkt hassas ayar baz alınıyor , x x1 y y1 de range aralıgnı tutturma fonksıyonunu dene yenı ayarladım."
      # "Bu bölüm, listbox öğelerini dinleme görevini üstlenir. \n\nKullanıcının seçtiği frekansların burada kodlaması yapılmıştır. \n\nEğer seçilen frekanslar için Excel’den veri varsa, bu veriler Excel dosyasından okunup ilgili alanlara aktarılır. \n\nAyrıca, interrupt (kesinti) denge koşulu ve manuel setup işlemleri (sadece Excel’deki değerlerin input olarak alınması) de bu kısımda gerçekleştirilir."
      # "X Series Sharing Reference Clock and \nMaster-Slave Trigger Synchronization \nfor PXIe Devices"
      # "Send Trigger"
      # "Acquire Data"
      # "Start Slave task before Master task"
      n121 = disable-structure shown="Disabled" {
        disable-tunnel: [w529 _] -> w62
        disable-tunnel: [w528 _] -> w61
        frame Disabled {
          w554 = 10097 items=["Allow Regeneration"=10097, "Do Not Allow Regeneration"=10158]  # regeneration mode
          w552 = 10123 items=["Finite Samples"=10178, "Continuous Samples"=10123, "Hardware Timed Single Point"=12522]  # sample mode
          w551 = 2000  # number of samples
          w550 = 204800.0  # rate
          w547 = 10106 items=["Default"=-1, "RSE"=10083, "Differential"=10106, "Pseudodifferential"=12529]  # output terminal configuration
          w546 = 10348 items=["Volts"=10348, "From Custom Scale"=10065]  # units
          w545 = "VoltageOut_1"  # channel name
          w543 = ""  # custom scale name
          w542 = -10.0  # minimum value
          w541 = 10.0  # maximum value
          (unwired) "Dev3/ao1"  # physical channel
          w539 = 10106 items=["Default"=-1, "RSE"=10083, "Differential"=10106, "Pseudodifferential"=12529]  # output terminal configuration
          w538 = 10348 items=["Volts"=10348, "From Custom Scale"=10065]  # units
          w537 = "VoltageOut_0"  # channel name
          w535 = ""  # custom scale name
          w534 = -10.0  # minimum value
          w533 = 10.0  # maximum value
          (unwired) "Dev3/ao0"  # physical channel
          w531 = TRUE  # auto cleanup
          n122 = call <vilib>:"DAQmx Create Task.vi"("auto cleanup"=w531) -> ("task out"=w532:refnum<k21>, "error out"=w530:errorcluster)  [unwired: 13 in]
          n123 = call-poly <vilib>:"DAQmx Create Virtual Channel.vi"("task in"=w532, "maximum value"=w533, "minimum value"=w534, "output terminal configuration"=w539, "physical channels"=tag "Dev3/ao0", "name to assign"=w537, "units"=w538, "error in"=w530, "custom scale name"=w535) -> ("task out"=w540:refnum<k21>, "error out"=w536:errorcluster)  [unwired: 5 in]
          n124 = call-poly <vilib>:"DAQmx Create Virtual Channel.vi"("task in"=w540, "maximum value"=w541, "minimum value"=w542, "output terminal configuration"=w547, "physical channels"=tag "Dev3/ao1", "name to assign"=w545, "units"=w546, "error in"=w536, "custom scale name"=w543) -> ("task out"=w549:refnum<k21>, "error out"=w544:errorcluster)  [unwired: 5 in]
          n125 = call-poly <vilib>:"DAQmx Timing.vi"("task/channels in"=w549, "sample mode"=w552, "samples per channel"=w551, "rate"=w550, "error in"=w544) -> ("task out"=w553:refnum<k21>, "error out"=w548:errorcluster)  [unwired: 9 in]
          n126 = property class="DAQmx Write"(reference=w553, error in=w548, "Regeneration Mode"=w554) -> (reference out=w529:refnum<k21>, error out=w528:errorcluster)
        }
        frame Enabled {
        }
      }
      n127 = call <vilib>:"DAQmx Create Task.vi"("auto cleanup"=w173) -> ("task out"=w172:refnum<k21>, "error out"=w174:errorcluster)  [unwired: 13 in]
      n128 = call <vilib>:"DAQmx Create Task.vi"("auto cleanup"=w176) -> ("task out"=w177:refnum<k21>, "error out"=w175:errorcluster)  [unwired: 13 in]
      n129 = call <vilib>:"DAQmx Create Task.vi"("auto cleanup"=w239) -> ("task out"=w238:refnum<k21>, "error out"=w240:errorcluster)  [unwired: 13 in]
      n130 = call <vilib>:"DAQmx Create Task.vi"("auto cleanup"=w329) -> ("task out"=w328:refnum<k21>, "error out"=w71:errorcluster)  [unwired: 13 in]
      n131 = disable-structure shown="Disabled" {
        disable-tunnel: w71 -> [w471 _]
        disable-tunnel: [w470 _] -> w70
        disable-tunnel: [w469 _] -> w69
        frame Disabled {
          w499 = 10123 items=["Finite Samples"=10178, "Continuous Samples"=10123, "Hardware Timed Single Point"=12522]  # sample mode
          w498 = 2000  # number of samples
          w497 = 204800.0  # rate
          w493 = 10045 items=["AC"=10045, "DC"=10050, "GND"=10066]  # Coupling
          w492 = "Voltage_1"  # ActiveChan
          w489 = 10045 items=["AC"=10045, "DC"=10050, "GND"=10066]  # Coupling
          w488 = "Voltage_0"  # ActiveChan
          w487 = 10106 items=["default"=-1, "RSE"=10083, "NRSE"=10078, "Differential"=10106, "Pseudodifferential"=12529]  # input terminal configuration
          w486 = 10348 items=["Volts"=10348, "From Custom Scale"=10065]  # units
          w485 = "Voltage_1"  # channel name
          w501 = ""  # custom scale name
          w483 = -10.0  # minimum value
          w482 = 10.0  # maximum value
          (unwired) "Dev3/ai1"  # physical channel
          w480 = 10106 items=["default"=-1, "RSE"=10083, "NRSE"=10078, "Differential"=10106, "Pseudodifferential"=12529]  # input terminal configuration
          w479 = 10348 items=["Volts"=10348, "From Custom Scale"=10065]  # units
          w478 = "Voltage_0"  # channel name
          w500 = ""  # custom scale name
          w476 = -10.0  # minimum value
          w475 = 10.0  # maximum value
          (unwired) "Dev3/ai0"  # physical channel
          w473 = TRUE  # auto cleanup
          n132 = call <vilib>:"DAQmx Create Task.vi"("auto cleanup"=w473, "error in"=w471) -> ("task out"=w474:refnum<k21>, "error out"=w472:errorcluster)  [unwired: 12 in]
          n133 = call-poly <vilib>:"DAQmx Create Virtual Channel.vi"("task in"=w474, "maximum value"=w475, "minimum value"=w476, "input terminal configuration"=w480, "physical channels"=tag "Dev3/ai0", "name to assign"=w478, "units"=w479, "error in"=w472, "custom scale name"=w500) -> ("task out"=w481:refnum<k21>, "error out"=w477:errorcluster)  [unwired: 5 in]
          n134 = call-poly <vilib>:"DAQmx Create Virtual Channel.vi"("task in"=w481, "maximum value"=w482, "minimum value"=w483, "input terminal configuration"=w487, "physical channels"=tag "Dev3/ai1", "name to assign"=w485, "units"=w486, "error in"=w477, "custom scale name"=w501) -> ("task out"=w491:refnum<k21>, "error out"=w484:errorcluster)  [unwired: 5 in]
          n135 = property class="DAQmx Channel"(reference=w491, error in=w484, "Active Channels (if subset)"=w488, "Analog Input:General Properties:Input Configuration:Coupling"=w489) -> (reference out=w495:refnum<k21>, error out=w490:errorcluster)
          n136 = property class="DAQmx Channel"(reference=w495, error in=w490, "Active Channels (if subset)"=w492, "Analog Input:General Properties:Input Configuration:Coupling"=w493) -> (reference out=w496:refnum<k21>, error out=w494:errorcluster)
          n137 = call-poly <vilib>:"DAQmx Timing.vi"("task/channels in"=w496, "sample mode"=w499, "samples per channel"=w498, "rate"=w497, "error in"=w494) -> ("task out"=w470:refnum<k21>, "error out"=w469:errorcluster)  [unwired: 9 in]
        }
        frame Enabled {
        }
      }
      n138 = call <vilib>:"DAQmx Create Task.vi"("auto cleanup"=w274, "error in"=w71) -> ("task out"=w275:refnum<k21>, "error out"=w273:errorcluster)  [unwired: 12 in]
      n139 = call-poly <vilib>:"DAQmx Create Virtual Channel.vi"("task in"=w172, "maximum value"=w171, "minimum value"=w170, "output terminal configuration"=w165, "physical channels"=tag "PXI1Slot2/ao0", "name to assign"=w167, "units"=w166, "error in"=w174, "custom scale name"=w169) -> ("task out"=w164:refnum<k21>, "error out"=w168:errorcluster)  [unwired: 5 in]
      n140 = call-poly <vilib>:"DAQmx Create Virtual Channel.vi"("task in"=w177, "maximum value"=w178, "minimum value"=w179, "output terminal configuration"=w184, "physical channels"=tag "Dev1/ao0", "name to assign"=w182, "units"=w183, "error in"=w175, "custom scale name"=w180) -> ("task out"=w185:refnum<k21>, "error out"=w181:errorcluster)  [unwired: 5 in]
      n141 = call <vilib>:"DAQmx Create Task.vi"("auto cleanup"=w271, "error in"=w71) -> ("task out"=w270:refnum<k21>, "error out"=w272:errorcluster)  [unwired: 12 in]
      n142 = call-poly <vilib>:"DAQmx Create Virtual Channel.vi"("task in"=w238, "maximum value"=w237, "minimum value"=w236, "output terminal configuration"=w231, "physical channels"=tag "Dev2/ao0", "name to assign"=w233, "units"=w232, "error in"=w240, "custom scale name"=w235) -> ("task out"=w230:refnum<k21>, "error out"=w234:errorcluster)  [unwired: 5 in]
      n143 = call-poly <vilib>:"DAQmx Create Virtual Channel.vi"("task in"=w164, "maximum value"=w163, "minimum value"=w162, "output terminal configuration"=w157, "physical channels"=tag "PXI1Slot2/ao1", "name to assign"=w159, "units"=w158, "error in"=w168, "custom scale name"=w161) -> ("task out"=w155:refnum<k21>, "error out"=w160:errorcluster)  [unwired: 5 in]
      n144 = call-poly <vilib>:"DAQmx Create Virtual Channel.vi"("task in"=w185, "maximum value"=w186, "minimum value"=w187, "output terminal configuration"=w192, "physical channels"=tag "Dev1/ao1", "name to assign"=w190, "units"=w191, "error in"=w181, "custom scale name"=w188) -> ("task out"=w194:refnum<k21>, "error out"=w189:errorcluster)  [unwired: 5 in]
      n145 = call-poly <vilib>:"DAQmx Create Virtual Channel.vi"("task in"=w275, "maximum value"=w276, "minimum value"=w277, "input terminal configuration"=w281, "physical channels"=tag "Dev1/ai0", "name to assign"=w279, "units"=w280, "error in"=w273, "custom scale name"=w244) -> ("task out"=w282:refnum<k21>, "error out"=w278:errorcluster)  [unwired: 5 in]
      n146 = call-poly <vilib>:"DAQmx Create Virtual Channel.vi"("task in"=w270, "maximum value"=w269, "minimum value"=w268, "input terminal configuration"=w264, "physical channels"=tag "Dev2/ai0", "name to assign"=w266, "units"=w265, "error in"=w272, "custom scale name"=w243) -> ("task out"=w263:refnum<k21>, "error out"=w267:errorcluster)  [unwired: 5 in]
      n147 = call-poly <vilib>:"DAQmx Create Virtual Channel.vi"("task in"=w328, "maximum value"=w327, "minimum value"=w326, "input terminal configuration"=w321, "physical channels"=tag "PXI1Slot2/ai0", "name to assign"=w323, "units"=w322, "error in"=w71, "custom scale name"=w325) -> ("task out"=w320:refnum<k21>, "error out"=w324:errorcluster)  [unwired: 5 in]
      n148 = call-poly <vilib>:"DAQmx Create Virtual Channel.vi"("task in"=w230, "maximum value"=w229, "minimum value"=w228, "output terminal configuration"=w223, "physical channels"=tag "Dev2/ao1", "name to assign"=w225, "units"=w224, "error in"=w234, "custom scale name"=w227) -> ("task out"=w221:refnum<k21>, "error out"=w226:errorcluster)  [unwired: 5 in]
      n149 = call-poly <vilib>:"DAQmx Timing.vi"("task/channels in"=w155, "sample mode"=w152, "samples per channel"=w153, "rate"=w154, "error in"=w160) -> ("task out"=w151:refnum<k21>, "error out"=w156:errorcluster)  [unwired: 9 in]
      n150 = call-poly <vilib>:"DAQmx Timing.vi"("task/channels in"=w194, "sample mode"=w197, "samples per channel"=w196, "rate"=w195, "error in"=w189) -> ("task out"=w198:refnum<k21>, "error out"=w193:errorcluster)  [unwired: 9 in]
      n151 = call-poly <vilib>:"DAQmx Timing.vi"("task/channels in"=w221, "sample mode"=w218, "samples per channel"=w219, "rate"=w220, "error in"=w226) -> ("task out"=w217:refnum<k21>, "error out"=w222:errorcluster)  [unwired: 9 in]
      n152 = call-poly <vilib>:"DAQmx Create Virtual Channel.vi"("task in"=w282, "maximum value"=w283, "minimum value"=w284, "input terminal configuration"=w288, "physical channels"=tag "Dev1/ai1", "name to assign"=w286, "units"=w287, "error in"=w278, "custom scale name"=w242) -> ("task out"=w292:refnum<k21>, "error out"=w285:errorcluster)  [unwired: 5 in]
      n153 = call-poly <vilib>:"DAQmx Create Virtual Channel.vi"("task in"=w263, "maximum value"=w262, "minimum value"=w261, "input terminal configuration"=w257, "physical channels"=tag "Dev2/ai1", "name to assign"=w259, "units"=w258, "error in"=w267, "custom scale name"=w241) -> ("task out"=w253:refnum<k21>, "error out"=w260:errorcluster)  [unwired: 5 in]
      n154 = call-poly <vilib>:"DAQmx Create Virtual Channel.vi"("task in"=w320, "maximum value"=w319, "minimum value"=w318, "input terminal configuration"=w313, "physical channels"=tag "PXI1Slot2/ai1", "name to assign"=w315, "units"=w314, "error in"=w324, "custom scale name"=w317) -> ("task out"=w309:refnum<k21>, "error out"=w316:errorcluster)  [unwired: 5 in]
      n155 = property class="DAQmx Write"(reference=w151, error in=w156, "Regeneration Mode"=w150) -> (reference out=w149:refnum<k21>, error out=w148:errorcluster)
      n156 = property class="DAQmx Write"(reference=w198, error in=w193, "Regeneration Mode"=w199) -> (reference out=w147:refnum<k21>, error out=w146:errorcluster)
      n157 = property class="DAQmx Write"(reference=w217, error in=w222, "Regeneration Mode"=w216) -> (reference out=w209:refnum<k21>, error out=w208:errorcluster)
      n158 = property class="DAQmx Channel"(reference=w292, error in=w285, "Active Channels (if subset)"=w289, "Analog Input:General Properties:Input Configuration:Coupling"=w290) -> (reference out=w296:refnum<k21>, error out=w291:errorcluster)
      n159 = property class="DAQmx Channel"(reference=w253, error in=w260, "Active Channels (if subset)"=w256, "Analog Input:General Properties:Input Configuration:Coupling"=w255) -> (reference out=w249:refnum<k21>, error out=w254:errorcluster)
      n160 = property class="DAQmx Channel"(reference=w309, error in=w316, "Active Channels (if subset)"=w312, "Analog Input:General Properties:Input Configuration:Coupling"=w311) -> (reference out=w305:refnum<k21>, error out=w310:errorcluster)
      n161 = property class="DAQmx Channel"(reference=w296, error in=w291, "Active Channels (if subset)"=w293, "Analog Input:General Properties:Input Configuration:Coupling"=w294) -> (reference out=w297:refnum<k21>, error out=w295:errorcluster)
      n162 = property class="DAQmx Channel"(reference=w249, error in=w254, "Active Channels (if subset)"=w252, "Analog Input:General Properties:Input Configuration:Coupling"=w251) -> (reference out=w248:refnum<k21>, error out=w250:errorcluster)
      n163 = property class="DAQmx Channel"(reference=w305, error in=w310, "Active Channels (if subset)"=w308, "Analog Input:General Properties:Input Configuration:Coupling"=w307) -> (reference out=w304:refnum<k21>, error out=w306:errorcluster)
      n164 = call-poly <vilib>:"DAQmx Timing.vi"("task/channels in"=w297, "sample mode"=w300, "samples per channel"=w299, "rate"=w298, "error in"=w295) -> ("task out"=w116:refnum<k21>, "error out"=w117:errorcluster)  [unwired: 9 in]
      n165 = call-poly <vilib>:"DAQmx Timing.vi"("task/channels in"=w248, "sample mode"=w245, "samples per channel"=w246, "rate"=w247, "error in"=w250) -> ("task out"=w115:refnum<k21>, "error out"=w114:errorcluster)  [unwired: 9 in]
      n166 = call-poly <vilib>:"DAQmx Timing.vi"("task/channels in"=w304, "sample mode"=w301, "samples per channel"=w302, "rate"=w303, "error in"=w306) -> ("task out"=w121:refnum<k21>, "error out"=w120:errorcluster)  [unwired: 9 in]
      n167 = global read "DB_Global_4_kart-Test.vi" "Input.BufSize"() -> (w68:u32)
      n168 = disable-structure shown="Disabled" {
        disable-tunnel: w70 -> [w468 _]
        disable-tunnel: w69 -> [w467 _]
        disable-tunnel: w68 -> [w466 _]
        disable-tunnel: [w465 _] -> w67
        disable-tunnel: [w464 _] -> w66
        frame Disabled {
          n169 = property class="DAQmx Buffer"(reference=w468, error in=w467, "Input:Buffer Size"=w466) -> (reference out=w465:refnum<k21>, error out=w464:errorcluster)
        }
